vi "Convert From XML Configuration File.vi"   [LabVIEW 2014]
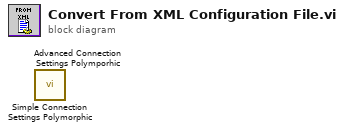
[diagram p0: block diagram]
diagram:
  n1 = call "Simple Connection Settings Polymorphic.vi"() -> ()  [unwired: 10 in, 2 out]
  n2 = call "Advanced Connection Settings Polymporhic.vi"() -> ()  [unwired: 10 in, 2 out]
